vi "smoothing FIR with delay.vi"(1 "delay":enum16{"1", "2", "3", "4", "5", "6", "7"}(ring), 7 "x in":dbl) -> (8 "x out":dbl)   [LabVIEW 2016]
doc: "this vi smooths data using a \"Gaussian\" averaging filter\n\nPaul K Dixon\nCSUSB Physics"
uses:
  <vilib>/ptbypt/NI_PtbyPt.lvlib
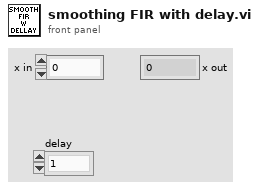
[diagram p1: front panel]
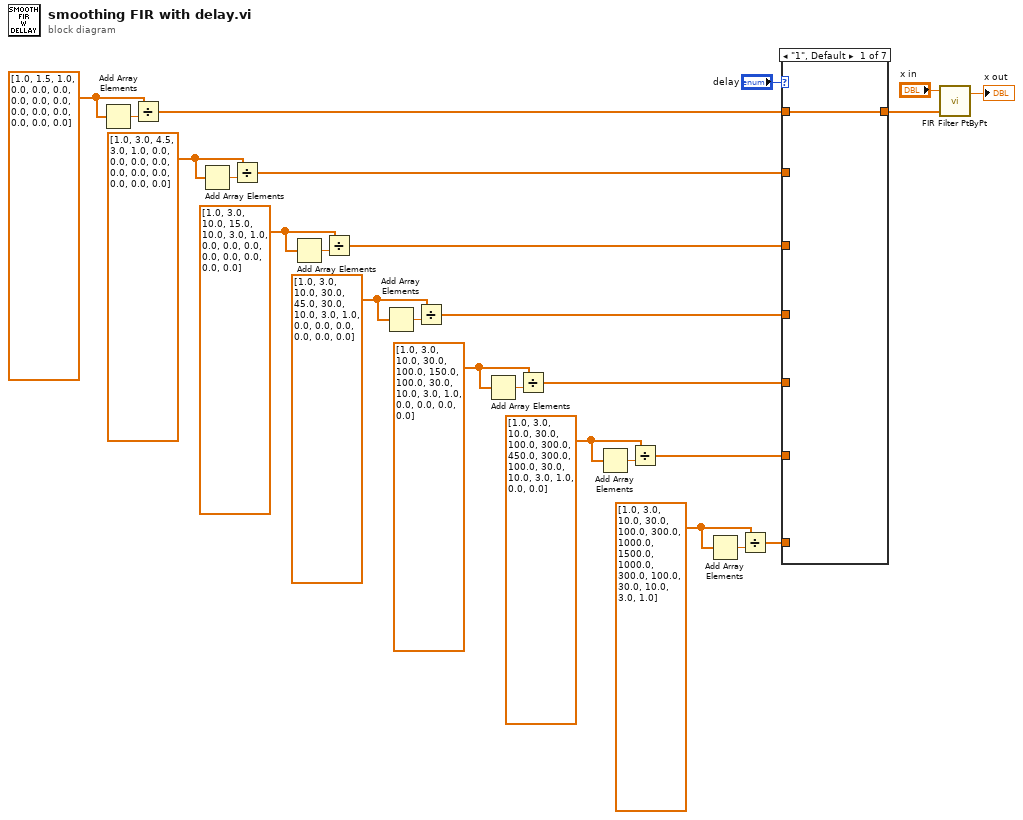
[diagram p0: block diagram]
diagram:
  w11 = dbl[] [1.0, 1.5, 1.0, 0.0, 0.0, 0.0, 0.0, 0.0, 0.0, 0.0, 0.0, 0.0, 0.0, 0.0, 0.0] ("Forward Coefficients")
  w12 = dbl[] [1.0, 3.0, 4.5, 3.0, 1.0, 0.0, 0.0, 0.0, 0.0, 0.0, 0.0, 0.0, 0.0, 0.0, 0.0] ("Forward Coefficients")
  w14 = dbl[] [1.0, 3.0, 10.0, 15.0, 10.0, 3.0, 1.0, 0.0, 0.0, 0.0, 0.0, 0.0, 0.0, 0.0, 0.0] ("Forward Coefficients")
  w16 = dbl[] [1.0, 3.0, 10.0, 30.0, 45.0, 30.0, 10.0, 3.0, 1.0, 0.0, 0.0, 0.0, 0.0, 0.0, 0.0] ("Forward Coefficients")
  w19 = dbl[] [1.0, 3.0, 10.0, 30.0, 100.0, 300.0, 1000.0, 1500.0, 1000.0, 300.0, 100.0, 30.0, 10.0, 3.0, 1.0] ("Forward Coefficients")
  w20 = dbl[] [1.0, 3.0, 10.0, 30.0, 100.0, 300.0, 450.0, 300.0, 100.0, 30.0, 10.0, 3.0, 1.0, 0.0, 0.0] ("Forward Coefficients")
  w25 = dbl[] [1.0, 3.0, 10.0, 30.0, 100.0, 150.0, 100.0, 30.0, 10.0, 3.0, 1.0, 0.0, 0.0, 0.0, 0.0] ("Forward Coefficients")
  # "1"
  # "2"
  # "3"
  # "4"
  # "7"
  # "6"
  # "5"
  n1 = Add Array Elements(numeric array=w11) -> (sum=w10:dbl)
  n2 = Divide(x=w11, y=w10) -> (x/y=w8:dbl[])
  n3 = Add Array Elements(numeric array=w12) -> (sum=w13:dbl)
  n4 = Divide(x=w12, y=w13) -> (x/y=w7:dbl[])
  n5 = Add Array Elements(numeric array=w14) -> (sum=w15:dbl)
  n6 = Divide(x=w14, y=w15) -> (x/y=w2:dbl[])
  n7 = Add Array Elements(numeric array=w16) -> (sum=w17:dbl)
  n8 = Divide(x=w16, y=w17) -> (x/y=w3:dbl[])
  n9 = Add Array Elements(numeric array=w25) -> (sum=w22:dbl)
  n10 = Divide(x=w25, y=w22) -> (x/y=w4:dbl[])
  n11 = Add Array Elements(numeric array=w20) -> (sum=w21:dbl)
  n12 = Divide(x=w20, y=w21) -> (x/y=w5:dbl[])
  n13 = Add Array Elements(numeric array=w19) -> (sum=w18:dbl)
  n14 = Divide(x=w19, y=w18) -> (x/y=w6:dbl[])
  n15 = case shown="\"1\", Default" "delay" {
    tunnel: w8 -> [w26 _ _ _ _ _ _]
    tunnel: w7 -> [_ w27 _ _ _ _ _]
    tunnel: w6 -> [_ _ _ _ _ _ w32]
    tunnel: w5 -> [_ _ _ _ _ w31 _]
    tunnel: w4 -> [_ _ _ _ w30 _ _]
    tunnel: w3 -> [_ _ _ w29 _ _ _]
    tunnel: w2 -> [_ _ w28 _ _ _ _]
    tunnel: [w26 w27 w28 w29 w30 w31 w32] -> w1
    frame "1", Default {
    }
    frame "2" {
    }
    frame "3" {
    }
    frame "4" {
    }
    frame "5" {
    }
    frame "6" {
    }
    frame "7" {
    }
  }
  n16 = call <vilib>:"FIR Filter PtByPt.vi"("Forward Coefficients"=w1, "x"="x in") -> ("Filtered x"=→"x out":dbl)  [unwired: 2 in, 1 out]
